vi "GSI-HVSwitch2.set channel voltage.vi"(0 "i ref in":refnum<vi>, 1 "nomVoltage":dbl format="%.2f", 2 "channel":i32, 3 "ms timeout (10000)":i32=10000, 5 "error in (no error)":errorcluster) -> (14 "i ref out":refnum<vi>, 17 "timed out":bool, 19 "error out":errorcluster)   [LabVIEW 2014, in "GSI-HVSwitch2.lvlib"]
doc: "Sets the nominal voltage of the instrument."
uses:
  GSI-HVSwitch2.lvlib
  CS_Core/CSApplicationBaseClasses/PSChannelBase/PSChannelBase.directionType.ctl
  CS_Core/CSApplicationBaseClasses/PSChannelBase/PSChannelBase.serviceType.ctl
  CSlibraries/UtilityLib/UtilityLib.valueStatus.ctl
  CS_Core/CSApplicationBaseClasses/DeviceBase/DeviceBase.deviceState.ctl
  CS_Core/CSSystem/CoreDefs/CoreDefs.error_type.ctl
  CS_Core/CSSystem/CoreDefs/CoreDefs.error_severity.ctl
  CS_Core/CSSystem/CoreLib/CoreLib.lvlib
  CS_Core/CSApplicationBaseClasses/PSChannelBase/PSChannelBase.lvlib
  CSlibraries/UtilityLib/UtilityLib.lvlib
  CS_Core/CSApplicationBaseClasses/DeviceBase/DeviceBase.lvlib
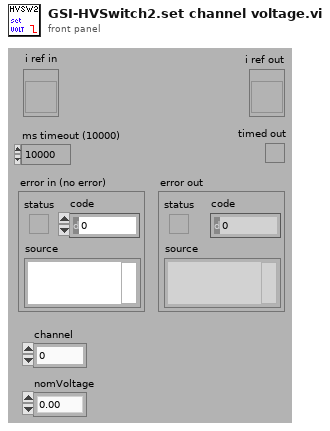
[diagram p1: front panel]
types:
  T1 = typedef "UtilityLib.lvlib/UtilityLib.valueStatus.ctl" = enum16{"no info available", "stand by/off", "on", "warning", "alarm/malfunction", "not implemented", "user action required", "important information", "system default", "control default", "indicator default", "button default"}
  T2 = typedef "PSChannelBase.lvlib/PSChannelBase.serviceType.ctl" = enum16{"onOff", "voltage", "current", "tripCurrent", "rampUpSpeed", "rampDownSpeed", "status"}
  T3 = typedef "PSChannelBase.lvlib/PSChannelBase.directionType.ctl" = enum16{"unknown", "update actual value", "update nominal value", "update both"}
  T4 = typedef "CoreDefs.error_severity.ctl" = enum16{"undefined", "information", "warning", "error", "fatal"}
  T5 = typedef "CoreDefs.error_type.ctl" = enum16{"no error", "can't load process", "can't unload process", "process does not exist", "can't install process", "can't remove process", "unknown function", "time out", "can't execute function", "duplicate queue name", "super not found", "caller queue invalid", "can't ping process", "unknown error", "VISA Error", "VISA timeout", "GPIB timeout", "GPIB error", "communication error", "data type mismatch", "can't read data from OPC server", "can't write data to OPC server", "OET error", "function not implemented", "process already exists", "invalid Shared Variable name", "error writing Shared Variable", "error reading Shared Variable", "invalid client name", "corrupt database", "unknown class", "call not authorized", "parameter out of range", "OET timeout: can't get data to modify", "invalid queue name", "requested operation incompatible with current state", "event undefined", "event disabled", "state undefined", "caller is not a friend", "EventBuilder: bad eventID", "EventBuilder: no DAQ devices", "a thread must not stop itself", "UNUSED ELEMENT4", "DiscArchiver: eventData incomplete", "DiscArchiver: eventData does not belong to run", "DiscArchiver: can't open file", "DiscArchiver: can't write to file", "DiscArchiver: available disc space low", "can't acquire semaphore", "error reading data from database", "notifier object is not existing", "can't register process", "can't unregister process", "illegal event type", "object disabled", "object already exists", "can't change state", "Instrument not found", "no connection to remote node", "invalid reference", "N/A", "UNUSED ELEMENT 1", "element not found", "illegal TCP/IP connection detected", "object does not exist", "invalid access ID", "unknown CS system", "invalid privilige", "unsupported data type", "unsupported server type", "IO server already exists", "Shared Variable already exists"}
  T6 = typedef "DeviceBase.lvlib/DeviceBase.deviceState.ctl" = i16
  T7 = typedef "GSI-HVSwitch2.lvlib/GSI-HVSwitch2.i attribute.ctl" = cluster{"SDEX VISA Cluster":T8, "SetVoltage SW0":dbl, "SetVoltage SW1":dbl, "ActTempAmp":dbl, "ActTempPS1":dbl, "ActTempPS2":dbl, "mode":T11, "interfaceInitialized":bool, "serviceIDs":cluster{"nomVoltage0ID":i32, "nomVoltage1ID":i32, "actTempAmpID":i32, "actTempPS1ID":i32, "actTempPS2ID":i32, "modeID":i32}, "usedChannels":i32}
  T8 = typedef "SDEXDriver.lvlib/SDEX.VISA Control.ctl" = cluster{"VISA resource name":refnum<visa-resource-name>, "HEX address":u16, "VISA Timeout Value (1000 ms)":u32, "Lock Timeout (1000 ms)":u32, "semaphore":T9, "Baud rate":u32, "revision":T10, "deviceInfo":string}
  T9 = typedef "Semaphore RefNum" = refnum<k1>
  T10 = typedef "SDEXDriver.lvlib/SDEX.revisionType.ctl" = enum16{"unknown", "hvamp3", "hvswi1", "htrp0", "WDG0"}
  T11 = typedef "GSI-HVSwitch2.lvlib/GSI-HVSwitch2.mode.ctl" = enum16{"unknown", "switch", "stepper"}
  T12 = typedef "PSChannelBase.lvlib/PSChannelBase.i attribute.ctl" = cluster{"defaultChannelIndex":i32, "nofChannels":i32, "defaultChannelIndexID":i32, "nofChannelsID":i32, "actValues":T13, "nomValues":T13, "logicalName":string[], "physicalName":string[], "logicalNameID":i32, "physicalNameID":i32}
  T13 = typedef "PSChannelBase.lvlib/PSChannelBase.parameters.ctl" = cluster{"onOff":bool[], "voltage":dbl[], "current":dbl[], "tripCurrent":dbl[], "rampUpSpeed":dbl[], "rampDownSpeed":dbl[], "status":i32[], "serviceIDs":cluster{"onOfflID":i32, "voltageID":i32, "currentID":i32, "tripCurrentID":i32, "rampUpSpeedID":i32, "rampDownSpeedID":i32, "statusID":i32}}
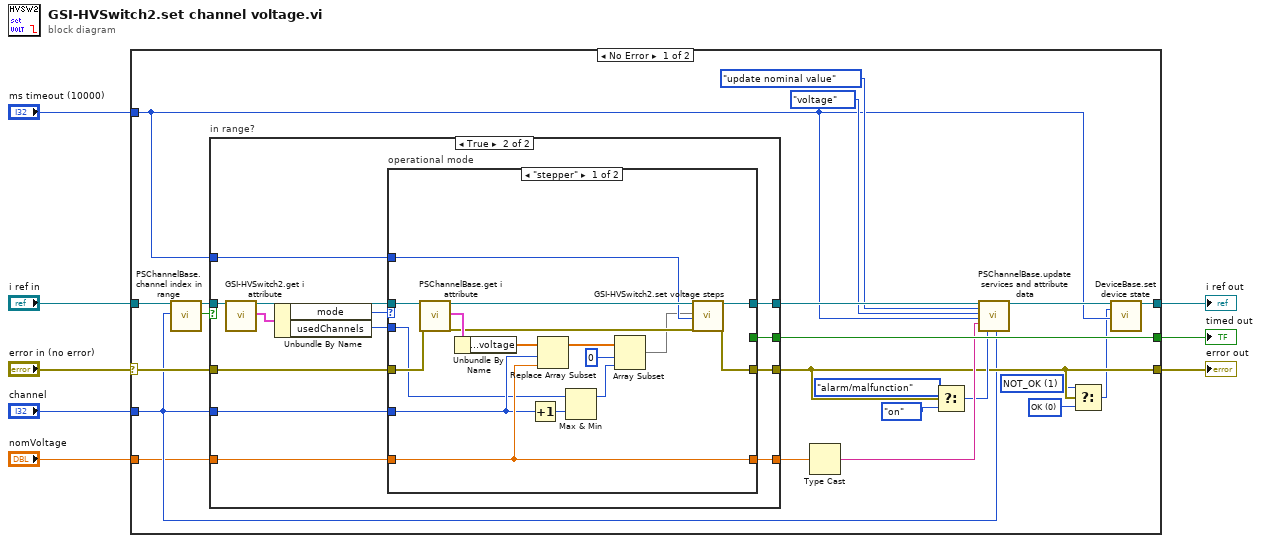
[diagram p0: block diagram]
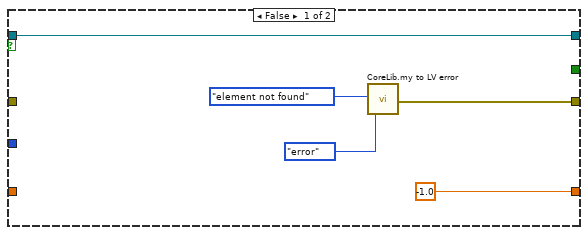
[diagram p2: hidden frame]
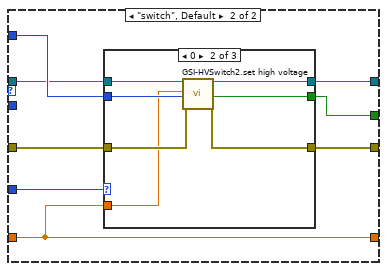
[diagram p3: hidden frame]
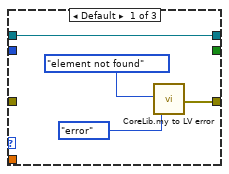
[diagram p4: hidden frame]
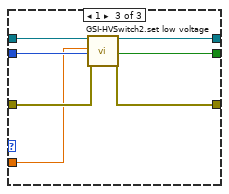
[diagram p5: hidden frame]
diagram:
  n1 = case shown="No Error" "error in (no error)" {
    selector: "error in (no error)" -> [w29 w92]
    tunnel: "i ref in" -> [w14 w93]
    tunnel: "ms timeout (10000)" -> [w19 _]
    tunnel: [w30 _] -> w6
    tunnel: [w20 w93] -> w5
    tunnel: [w18 w92] -> w4
    tunnel: "channel" -> [w11 _]
    tunnel: "nomVoltage" -> [w10 _]
    frame No Error {
      w16 = T6 1 items=["ERROR"=-1, "OK"=0, "NOT_OK"=1] ("deviceState")
      w17 = T6 0 items=["ERROR"=-1, "OK"=0, "NOT_OK"=1] ("deviceState")
      n2 = call "PSChannelBase.channel index in range.vi"("i ref in"=w14, "channelIndex"=w11) -> ("i ref out"=w13:refnum<vi>, "in range"=w12:bool)  [unwired: 15 in, 1 out]
      n3 = case "in range?" shown="True" w12 {
        tunnel: w13 -> [w33 w41]
        tunnel: w19 -> [_ w48]
        tunnel: [_ w47] -> w30
        tunnel: [w33 w44] -> w28
        tunnel: [w32 w46] -> w18
        tunnel: w29 -> [_ w45]
        tunnel: w11 -> [_ w43]
        tunnel: w10 -> [_ w42]
        tunnel: [-1.0 ("nomVoltage") w37] -> w9
        frame False {
          n4 = call "CoreLib.my to LV error.vi"("ErrorTypes"=CoreDefs.error_type."element not found", "severityLevel"=CoreDefs.error_severity."error") -> ("myErrorCluster"=w32:errorcluster)  [unwired: 16 in, 1 out]
        }
        frame True {
          n5 = call "GSI-HVSwitch2.get i attribute.vi"("i ref in"=w41) -> ("i ref out"=w38:refnum<vi>, "i attribute"=w40:T7)  [unwired: 16 in, 1 out]
          n6 = Unbundle By Name(w40) -> ("mode"=w39:T11, "usedChannels"=w36:i32)
          n7 = case "operational mode" shown="\"stepper\"" w39 {
            tunnel: w48 -> [w57 w73]
            tunnel: [_ w72] -> w47
            tunnel: [w55 w71] -> w46
            tunnel: w45 -> [w61 w70]
            tunnel: [w54 w69] -> w44
            tunnel: w43 -> [w52 w68]
            tunnel: w42 -> [w63 w66]
            tunnel: w38 -> [w62 w67]
            tunnel: [w63 w66] -> w37
            tunnel: w36 -> [w50 _]
            frame "stepper" {
              n8 = call "PSChannelBase.get i attribute.vi"("i ref in"=w62, "error in (no error)"=w61) -> ("i ref out"=w60:refnum<vi>, "i attribute"=w65:T12, "error out"=w56:errorcluster)  [unwired: 15 in]
              n9 = Unbundle By Name(w65) -> ("nomValues.voltage"=w64:dbl[])
              n10 = Increment(x=w52) -> (x+1=w51:i32)
              n11 = Replace Array Subset(array=w64, new element=w63, index=w52) -> (w59:dbl[])
              n12 = Max & Min(x=w50, y=w51) -> (max(x,y)=w49:i32)  [unwired: 1 out]
              n13 = Array Subset(array=w59, index=0, length=w49) -> (w53:dbl[])
              n14 = call "GSI-HVSwitch2.set voltage steps.vi"("i ref in"=w60, "voltageSteps [V]"=w53, "ms timeout (10000)"=w57, "error in (no error)"=w56) -> ("i ref out"=w54:refnum<vi>, "error out"=w55:errorcluster)  [unwired: 13 in, 1 out]
            }
            frame "switch", Default {
              n15 = case shown="0" w68 {
                tunnel: w67 -> [w77 w84 w91]
                tunnel: w73 -> [_ w79 w86]
                tunnel: [_ w83 w90] -> w72
                tunnel: [w75 w82 w89] -> w71
                tunnel: w70 -> [_ w81 w88]
                tunnel: [w77 w80 w87] -> w69
                tunnel: w66 -> [_ w78 w85]
                frame Default {
                  n16 = call "CoreLib.my to LV error.vi"("ErrorTypes"=CoreDefs.error_type."element not found", "severityLevel"=CoreDefs.error_severity."error") -> ("myErrorCluster"=w75:errorcluster)  [unwired: 16 in, 1 out]
                }
                frame 0 {
                  n17 = call "GSI-HVSwitch2.set high voltage.vi"("i ref in"=w84, "High Voltage"=w78, "ms timeout (10000)"=w79, "error in (no error)"=w81) -> ("i ref out"=w80:refnum<vi>, "timed out"=w83:bool, "error out"=w82:errorcluster)  [unwired: 13 in]
                }
                frame 1 {
                  n18 = call "GSI-HVSwitch2.set low voltage.vi"("i ref in"=w91, "Low Voltage"=w85, "ms timeout (10000)"=w86, "error in (no error)"=w88) -> ("i ref out"=w87:refnum<vi>, "timed out"=w90:bool, "error out"=w89:errorcluster)  [unwired: 13 in]
                }
              }
            }
          }
        }
      }
      n19 = Type Cast(x=w9) -> (*(type *) &x=w25:string)  [unwired: 1 in]
      n20 = Select(t=UtilityLib.valueStatus."alarm/malfunction" ("quality"), s=w18, f=UtilityLib.valueStatus."on") -> (s? t:f=w22:T1)
      n21 = call "PSChannelBase.update services and attribute data.vi"("i ref in"=w28, "direction"=PSChannelBase.directionType."update nominal value", "service"=PSChannelBase.serviceType."voltage", "ms timeout (10000)"=w19, "value"=w25, "quality"=w22, "channelNumber"=w11) -> ("i ref out"=w21:refnum<vi>)  [unwired: 10 in, 2 out]
      n22 = Select(t=w16, s=w18, f=w17) -> (s? t:f=w15:T6)
      n23 = call "DeviceBase.set device state.vi"("i ref in"=w21, "deviceState"=w15, "ms timeout (10000)"=w19) -> ("i ref out"=w20:refnum<vi>)  [unwired: 14 in, 2 out]
    }
    frame Error {
    }
  }
  "error out" <- w4
  "i ref out" <- w5
  "timed out" <- w6
